vi "Table Constructor Adv Schema DB.vi"(7 "Defer Constructor (F)":bool, 8 "error in (no error)":errorcluster, 9 "Table Name":string, 10 "Database":refnum<class "Database Adv Schema.lvclass">, 11 "Table Configuration Adv Schema DB in":refnum<class "Table Configuration Adv Schema DB.lvclass">) -> (0 "error out":errorcluster, 3 "Table Configuration Adv Schema DB out":refnum<class "Table Configuration Adv Schema DB.lvclass">)   [LabVIEW 2020, in "Table.lvlib" / "Table Configuration Adv Schema DB.lvclass"]
uses:
  Table Configuration Adv Schema DB.lvclass
  C:/Users/User/Desktop/Raman Program/Database OOP/source/Database OOP/Table Libraries/Basic Table/Configuration/Table Configuration Class/Table Configuration.lvclass
  Database Libraries/Database Interfaces/Database Advanced Schema Class/Database Adv Schema.lvclass
  Table Configuration Adv Schema DB.lvclass/Table Configuration Adv Schema DB.ctl
  Table Configuration Class/Table Configuration.lvclass/Table Configuration.ctl
  Table Configuration Class/Table Configuration.lvclass
panel:
  # "WARNING: deferring the constructor requires that you manaully call the constructor.vi method before accessing member data outside of the table configuration class!"
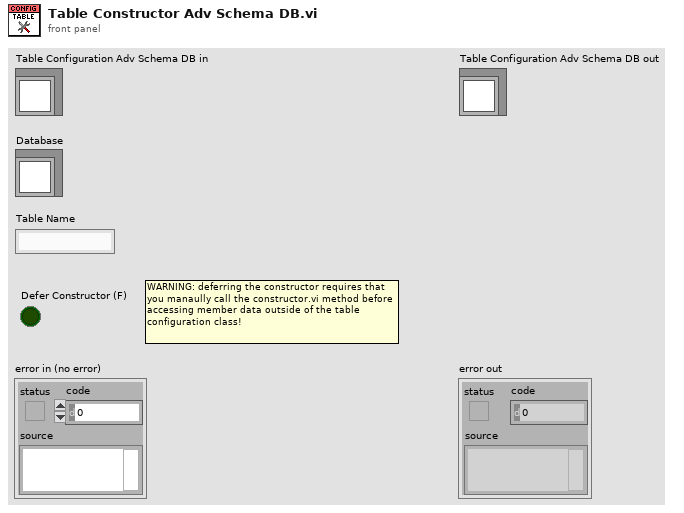
[diagram p1: front panel]
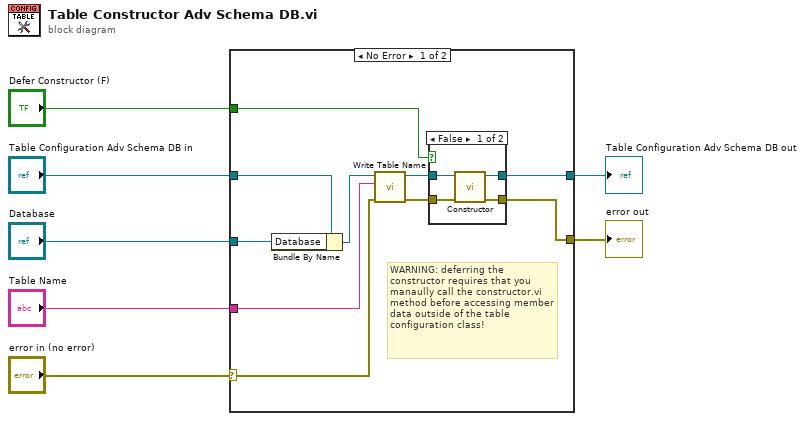
[diagram p0: block diagram]
diagram:
  n1 = case shown="No Error" "error in (no error)" {
    selector: "error in (no error)" -> [w9 w25]
    tunnel: [w10 w25] -> w6
    tunnel: [w11 w24] -> w4
    tunnel: "Table Configuration Adv Schema DB in" -> [w16 w24]
    tunnel: "Database" -> [w17 _]
    tunnel: "Table Name" -> [w14 _]
    tunnel: "Defer Constructor (F)" -> [w8 _]
    frame No Error {
      # "WARNING: deferring the constructor requires that you manaully call the constructor.vi method before accessing member data outside of the table configuration class!"
      n2 = Bundle By Name(cluster=w16, "Database"=w17) -> (w15:refnum<class "Table Configuration Adv Schema DB.lvclass">)
      n3 = call "Write Table Name.vi"("error in (no error)"=w9, "Table Name"=w14, "Table Configuration in"=w15) -> ("error out"=w12:errorcluster, "Table Configuration out"=w13:refnum<class "Table Configuration Adv Schema DB.lvclass">)  [unwired: 7 in]
      n4 = case shown="False" w8 {
        tunnel: w13 -> [w21 w23]
        tunnel: w12 -> [w20 w22]
        tunnel: [w19 w23] -> w11
        tunnel: [w18 w22] -> w10
        frame False {
          n5 = call-dynamic "Constructor.vi"("error in (no error)"=w20, "Table Configuration Adv Schema DB in"=w21) -> ("error out"=w18:errorcluster, "Table Configuration Adv Schema DB out"=w19:refnum<class "Table Configuration Adv Schema DB.lvclass">)  [unwired: 8 in]
        }
        frame True {
        }
      }
    }
    frame Error {
    }
  }
  "error out" <- w6
  "Table Configuration Adv Schema DB out" <- w4
